vi "cm2nm_new_session_dialog.vi"(8 "Notes":string, 9 "Session File":path, 10 "Session Name/ID":string, 11 "Instrument":T1) -> (0 "Session File_out":path, 1 "Session Name/ID_out":string, 2 "Notes_out":string, 3 "Instrument_out":u16)   [LabVIEW 2011]
doc: "Pressing the New Session with This Sample button opens up a dialog box to name and create a new file to store information about a new session. This dialog box requires a unique session name be entered in the Session Name/ID field before the OK button is enabled for the user to press. The user has the option to enter notes about the new session in a text box. The user also chooses an instrument type. The cancel button will abort the new session creation and return the program to the previous current session."
uses:
  Instrument_type_enum.ctl
panel:
  out "Session_path":path
  in  "Cancel":bool
  in  "OK Button":bool
  # "Instructions To Start a New Session\n1. Select instrument from drop list\n2. Enter a name or ID for the Session\n3. Optional: Enter notes about session more can be entered later in the session.\n4. Click OK button to start new session\nor cancel"
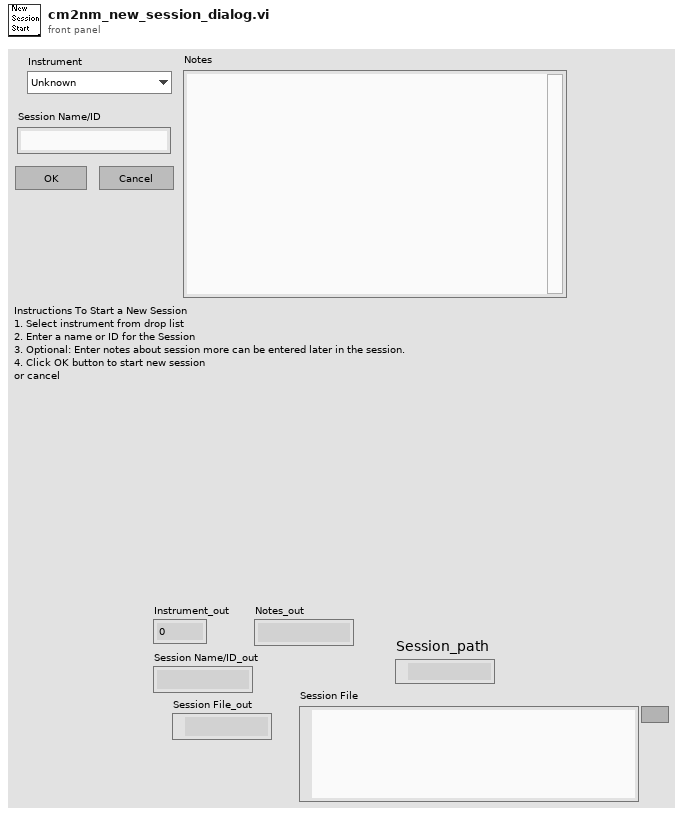
[diagram p1: front panel]
types:
  T1 = typedef "Instrument_type_enum.ctl" = enum16{"Unknown", "Phillips FEI SEM IRC", "JEOL 7000F EML_MFC", "MXRD MFC", "JEOL_EPMA"}
  T2 = enum8{"Enabled", "Disabled", "Disabled and Grayed Out"}
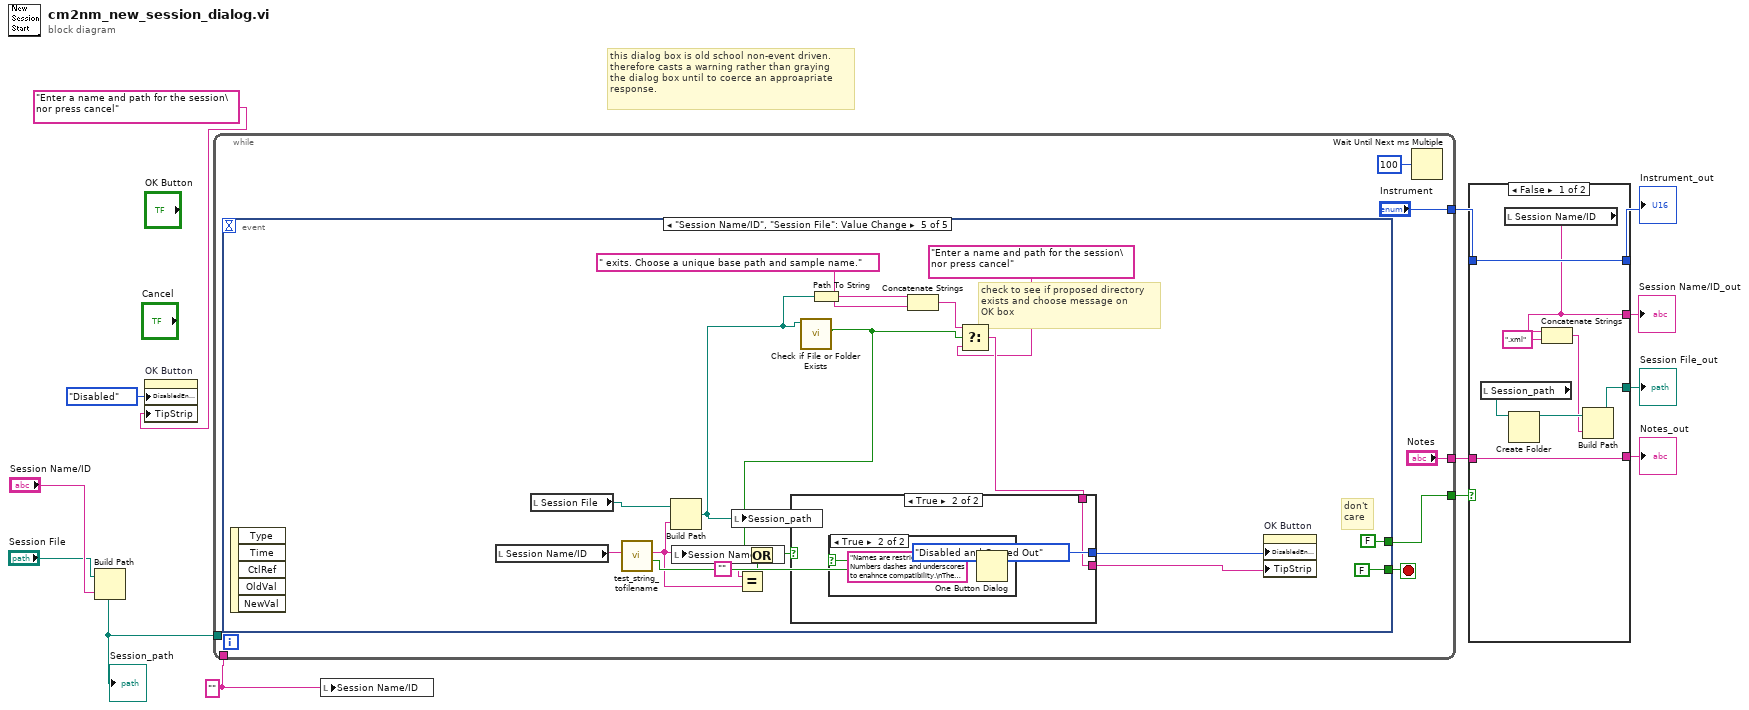
[diagram p0: block diagram]
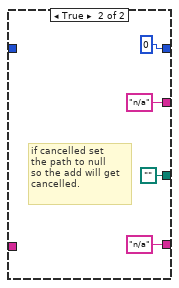
[diagram p2: hidden frame]
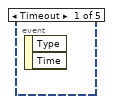
[diagram p3: hidden frame]
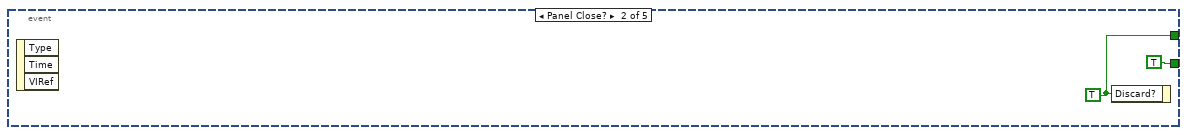
[diagram p4: hidden frame]
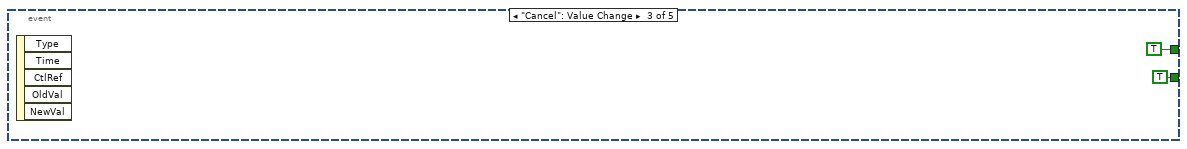
[diagram p5: hidden frame]
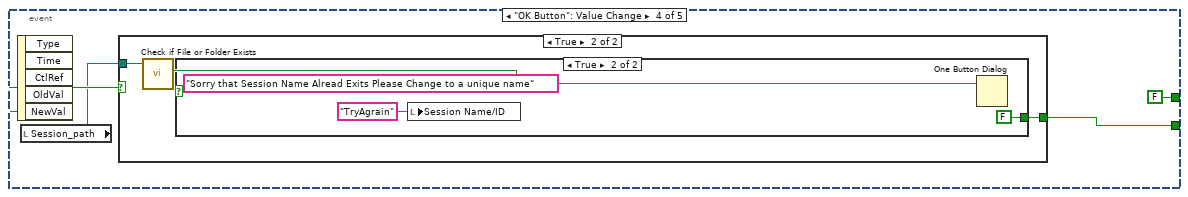
[diagram p6: hidden frame]
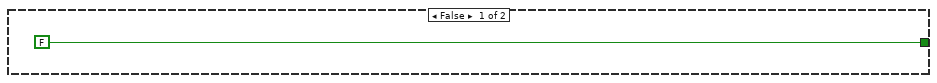
[diagram p7: hidden frame]
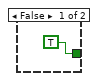
[diagram p8: hidden frame]
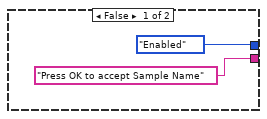
[diagram p9: hidden frame]
diagram:
  w6 = "" ("Session Name/ID")
  # "this dialog box is old school non-event driven.\ntherefore casts a warning rather than graying\nthe dialog box until to coerce an approapriate\nresponse."
  n1 = Build Path(base path="Session File", name or relative path="Session Name/ID") -> (appended path=w3:path)
  "Session_path" <- w3
  n2 = property on="OK Button" class="Bool"("DisabledEnum"=T2."Disabled" ("Disabled"), "TipStrip"="Enter a name and path for the session\nor press cancel" ("Tip Strip")) -> ()  [unwired: 2 in, 2 out]
  n3 = while {
    tunnel: ["Instrument"] -> w12
    tunnel: ["Notes"] -> w9
    tunnel: [w15] -> w13
    tunnel: w6 -> [_]
    tunnel: w3 -> [_]
    stop <- w14 stop-if-true
    n4 = event shown="[4] \"Session Name/ID\", \"Session File\": Value Change" {
      selector: _ -> [_ _ _ _ _]
      dyn-events: _ -> [_ _ _ _ _]
      timeout: _ -> [_ _ _ _ _]
      tunnel: [_ w20 TRUE ("Discard?") FALSE ("Discard?") FALSE ("Discard?")] -> w15
      tunnel: [_ TRUE TRUE w24 FALSE] -> w14
      event Timeout {
        n5 = event-data() -> ()  [unwired: 1 in, 2 out]
      }
      event Panel Close? {
        w20 = TRUE ("Discard?")
        n6 = event-data() -> ()  [unwired: 1 in, 3 out]
        n7 = event-data("Discard?"=w20) -> ()  [unwired: 1 in, 1 out]
      }
      event "Cancel": Value Change {
        n8 = event-data() -> ()  [unwired: 1 in, 5 out]
      }
      event "OK Button": Value Change {
        n9 = event-data() -> ("NewVal"=w26:bool)  [unwired: 1 in, 4 out]
        n10 = local read "Session_path"() -> (w25:path)
        n11 = case shown="True" w26 {
          tunnel: [FALSE w28] -> w24
          tunnel: w25 -> [_ w30]
          frame False {
          }
          frame True {
            n12 = call <vilib>:"Check if File or Folder Exists.vi"("path"=w30) -> ("file or folder exists?"=w29:bool)  [unwired: 8 in, 2 out]
            n13 = case shown="True" w29 {
              tunnel: [TRUE FALSE] -> w28
              frame False {
              }
              frame True {
                n14 = local write "Session Name/ID"("TryAgrain" ("Session Name/ID")) -> ()
                n15 = One Button Dialog(message="Sorry that Session Name Alread Exits Please Change to a unique name") -> ()  [unwired: 1 in, 1 out]
              }
            }
          }
        }
      }
      event "Session Name/ID", "Session File": Value Change {
        # "check to see if proposed directory\nexists and choose message on \nOK box"
        # "don't\ncare"
        n16 = event-data() -> ()  [unwired: 1 in, 5 out]
        n17 = local read "Session Name/ID"() -> (w49:string)
        n18 = local read "Session File"() -> (w52:path)
        n19 = call "test_string_tofilename.vi"("Session Name/ID"=w49) -> ("fixed_name"=w48:bool, "CompliantName"=w38:string)  [unwired: 9 in]
        n20 = Build Path(base path=w52, name or relative path=w38) -> (appended path=w39:path)
        n21 = local write "Session Name/ID"(w38) -> ()
        n22 = local write "Session_path"(w39) -> ()
        n23 = Equal?(x="", y=w38) -> (x = y?=w45:bool)
        n24 = call <vilib>:"Check if File or Folder Exists.vi"("path"=w39) -> ("file or folder exists?"=w42:bool)  [unwired: 8 in, 2 out]
        n25 = Or(x=w42, y=w45) -> (x .or. y?=w46:bool)
        n26 = Path To String(path=w39) -> (string=w44:string)
        n27 = case shown="True" w48 {
          frame False {
          }
          frame True {
            n28 = One Button Dialog(message="Names are restricted to Letters Numbers dashes and underscores to enahnce compatibility.\nThe name entered has been modified Please check it.") -> ()  [unwired: 1 in, 1 out]
          }
        }
        n29 = Concatenate Strings(w44, " exits. Choose a unique base path and sample name." ("string")) -> (w41:string)
        n30 = Select(t=w41, s=w42, f="Enter a name and path for the session\nor press cancel" ("Tip Strip")) -> (s? t:f=w40:string)
        n31 = case shown="True" w46 {
          tunnel: [T2."Enabled" ("Disabled") T2."Disabled and Grayed Out" ("Disabled")] -> w37
          tunnel: ["Press OK to accept Sample Name" ("Tip Strip") w55] -> w36
          tunnel: w40 -> [_ w55]
          frame False {
          }
          frame True {
          }
        }
        n32 = property on="OK Button" class="Bool"("DisabledEnum"=w37, "TipStrip"=w36) -> ()  [unwired: 2 in, 2 out]
      }
    }
    n33 = Wait Until Next ms Multiple(millisecond multiple=u32 100) -> ()  [unwired: 1 out]
  }
  n34 = local write "Session Name/ID"(w6) -> ()
  n35 = case shown="False" w13 {
    tunnel: w12 -> [w65 _]
    tunnel: [w65 u16 0 ("Instrument")] -> w11
    tunnel: [w59 "n/a" ("Session Name/ID")] -> w10
    tunnel: [w60 path ""] -> w8
    tunnel: [w64 "n/a" ("Notes")] -> w7
    tunnel: w9 -> [w64 _]
    frame False {
      n36 = local read "Session_path"() -> (w58:path)
      n37 = local read "Session Name/ID"() -> (w59:string)
      n38 = Create Folder(path (use dialog)=w58) -> (created path=w63:path)  [unwired: 2 in, 2 out]
      n39 = Concatenate Strings(w59, ".xml" ("string")) -> (w61:string)
      n40 = Build Path(base path=w63, name or relative path=w61) -> (appended path=w60:path)
    }
    frame True {
      # "if cancelled set\nthe path to null\nso the add will get \ncancelled."
    }
  }
  "Instrument_out" <- w11
  "Session Name/ID_out" <- w10
  "Session File_out" <- w8
  "Notes_out" <- w7
